vi "TableFinalizerRole.vi"(6 "Tactic index in":i32, 7 "first call":bool, 8 "error in (no error)":errorcluster, 10 "Game in":refnum<class "Game.lvclass">, 11 "TableFinalizerRole in":refnum<class "TableFinalizerRole.lvclass">) -> (0 "error out":errorcluster, 1 "tactic index":i32, 2 "Robot out":refnum<class "Robot.lvclass">, 3 "TableFinalizerRole out":refnum<class "TableFinalizerRole.lvclass">)   [LabVIEW 2023, in "TableFinalizerRole.lvclass"]
uses:
  TableFinalizerRole.lvclass
  Game_class/Game.lvclass
  Robot_class/Robot.lvclass
  Role_class/Role.lvclass/Role.ctl
  TableFinalizerRole.lvclass/TableFinalizerRole.ctl
  Tacticbook_class/Tacticbook.lvclass/Tacticbook.ctl
  TableReceiverTactic_class/TableReceiverTactic.lvclass/TableReceiverTactic.ctl
  ShootTactic_class/States.ctl
  ShootTactic_class/ShootTactic.lvclass/ShootTactic.ctl
  Tacticbook_class/Read TableReceiverTactic.vi
  TableReceiverTactic_class/Read States.vi
  Tacticbook_class/Write TableReceiverTactic.vi
  Tacticbook_class/Read WaitPassTactic.vi
  Tacticbook_class/Write WaitPassTactic.vi
  Tacticbook_class/Read ShootTactic.vi
  ShootTactic_class/Read States.vi
  Tacticbook_class/Write ShootTactic.vi
  Role_class/Read Tacticbook.vi
  Read number_of_tactics.vi
  Role_class/Write Tacticbook.vi
  Role_class/Write tactic_index.vi
  Role_class/Read RobotRef.vi
  Tacticbook_class/Tacticbook.lvclass
  KickToPassReceiverTactic_class/KickToPassReceiverTactic.lvclass
  TableReceiverTactic_class/TableReceiverTactic.lvclass
  WaitPassTactic_class/WaitPassTactic.lvclass
  ShootTactic_class/ShootTactic.lvclass
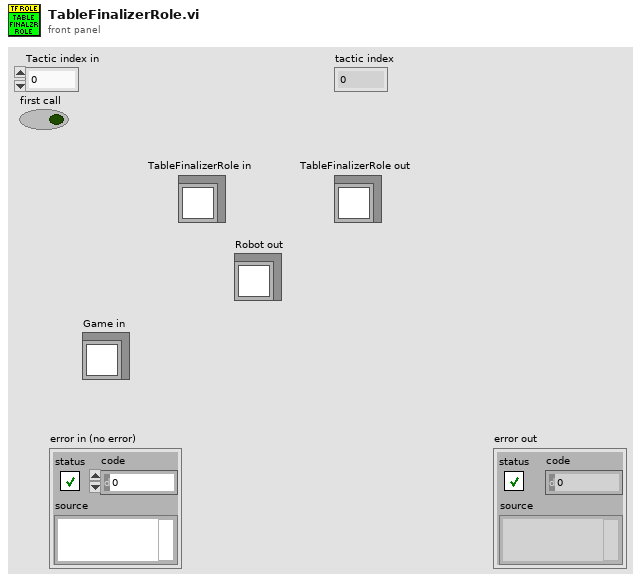
[diagram p1: front panel]
types:
  T1 = typedef "ShootTactic.lvclass/States.ctl" = enum16{"BallInGoalieArea", "Exit", "KickToGoal", "StealBall"}
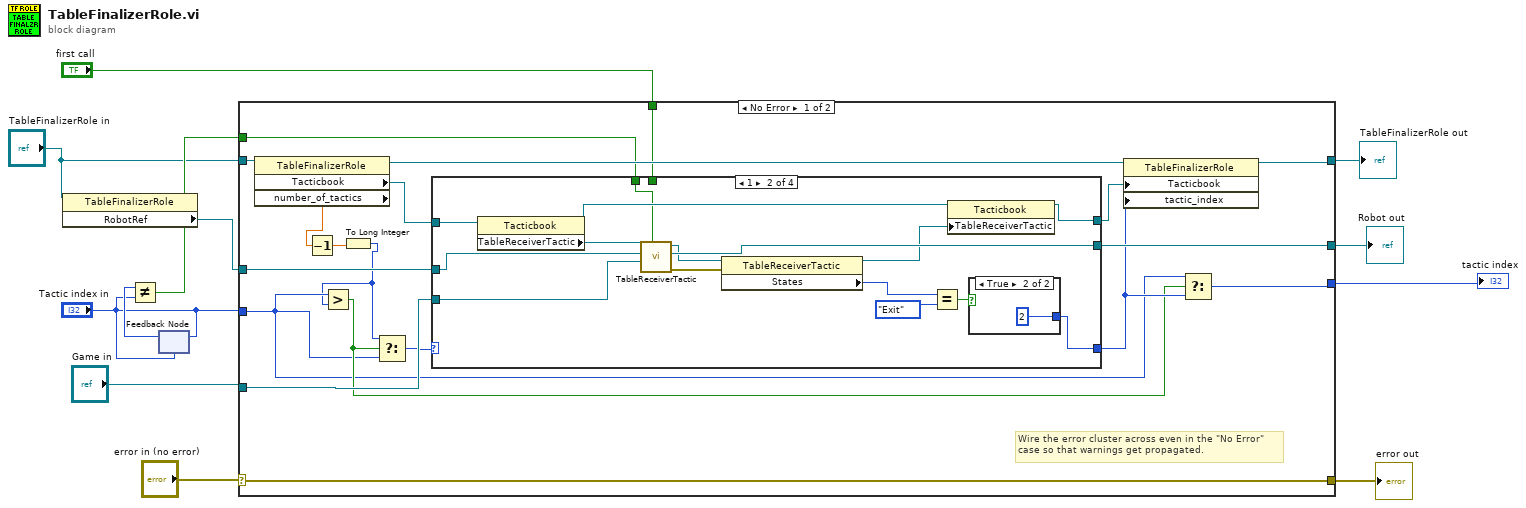
[diagram p0: block diagram]
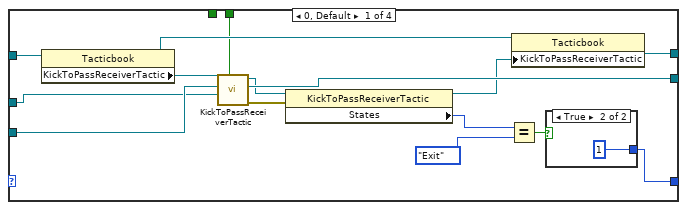
[diagram p2: hidden frame]
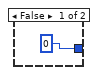
[diagram p3: hidden frame]
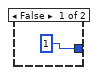
[diagram p4: hidden frame]
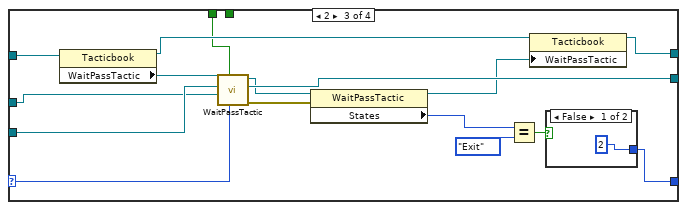
[diagram p5: hidden frame]
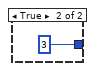
[diagram p6: hidden frame]
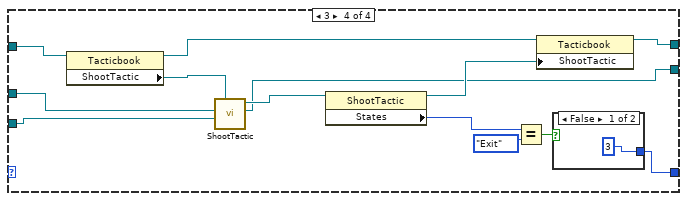
[diagram p7: hidden frame]
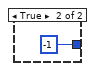
[diagram p8: hidden frame]
diagram:
  n1 = property class="TableFinalizerRole"(reference="TableFinalizerRole in") -> ("RobotRef"=w10:refnum<class "Robot.lvclass">)  [unwired: 1 in, 2 out]
  n2 = feedback #1("Tactic index in") -> (w6:i32)
  n3 = Not Equal?(x=w6, y="Tactic index in") -> (x != y?=w4:bool)
  n4 = feedback-in #1("Tactic index in") -> ()
  n5 = case shown="No Error" "error in (no error)" {
    selector: "error in (no error)" -> [w31 w101]
    tunnel: [w31 w101] -> w11
    tunnel: [w29 w100] -> w1
    tunnel: "TableFinalizerRole in" -> [w30 w100]
    tunnel: w10 -> [w26 w99]
    tunnel: [w25 w99] -> w3
    tunnel: "Game in" -> [w23 _]
    tunnel: [w21 _] -> w9
    tunnel: "Tactic index in" -> [w18 _]
    tunnel: "first call" -> [w16 _]
    tunnel: w4 -> [w13 _]
    frame No Error {
      # "Wire the error cluster across even in the \"No Error\"\ncase so that warnings get propagated."
      n6 = property class="TableFinalizerRole"(reference=w30) -> (reference out=w28:refnum<class "TableFinalizerRole.lvclass">, "Tacticbook"=w27:refnum<class "Tacticbook.lvclass">, "number_of_tactics"=w17:dbl)  [unwired: 1 in, 1 out]
      n7 = Decrement(x=w17) -> (x-1=w15:dbl)
      n8 = To Long Integer(number=w15) -> (32bit integer=w14:i32)
      n9 = Greater?(x=w18, y=w14) -> (0:w19:bool)
      n10 = Select(t=w14, s=w19, f=w18) -> (s? t:f=w20:i32)
      n11 = case shown="1" w20 {
        selector: w20 -> [_ _ w66 _]
        tunnel: [w34 w51 w69 w85] -> w22
        tunnel: w27 -> [w46 w63 w81 w94]
        tunnel: w26 -> [w37 w54 w72 w87]
        tunnel: [w45 w62 w80 w88] -> w25
        tunnel: [w41 w58 w76 w92] -> w24
        tunnel: w23 -> [w38 w55 w73 w86]
        tunnel: w16 -> [w32 _ _ _]
        tunnel: w13 -> [_ w49 w68 _]
        frame 0, Default {
          n12 = property class="Tacticbook"(reference=w46) -> (reference out=w43:refnum<class "Tacticbook.lvclass">, "KickToPassReceiverTactic"=w40:refnum<class "KickToPassReceiverTactic.lvclass">)  [unwired: 1 in, 1 out]
          n13 = call "KickToPassReceiverTactic.vi"("first call"=w32, "Robot"=w37, "Game in"=w38, "KickToPassReceiverTactic in"=w40) -> ("error out"=w44:errorcluster, "Robot out"=w45:refnum<class "Robot.lvclass">, "KickToPassReceiverTactic out"=w39:refnum<class "KickToPassReceiverTactic.lvclass">)  [unwired: 5 in]
          n14 = property class="KickToPassReceiverTactic"(reference=w39, error in=w44) -> (reference out=w42:refnum<class "KickToPassReceiverTactic.lvclass">, "States"=w35:enum16{"KickToPassReceiver", "WaitPass", "Exit"})  [unwired: 1 out]
          n15 = Equal?(x=w35, y=enum16{"KickToPassReceiver", "WaitPass", "Exit"}."Exit") -> (x = y?=w36:bool)
          n16 = property class="Tacticbook"(reference=w43, "KickToPassReceiverTactic"=w42) -> (reference out=w41:refnum<class "Tacticbook.lvclass">)  [unwired: 1 in, 1 out]
          n17 = case shown="True" w36 {
            tunnel: [0 1] -> w34
            frame False {
            }
            frame True {
            }
          }
        }
        frame 1 {
          n18 = property class="Tacticbook"(reference=w63) -> (reference out=w60:refnum<class "Tacticbook.lvclass">, "TableReceiverTactic"=w57:refnum<class "TableReceiverTactic.lvclass">)  [unwired: 1 in, 1 out]
          n19 = call "TableReceiverTactic.vi"("Firstcall?"=w49, "Game in"=w55, "Robot"=w54, "TableReceiverTactic in"=w57) -> ("error out"=w61:errorcluster, "Robot out"=w62:refnum<class "Robot.lvclass">, "TableReceiverTactic out"=w56:refnum<class "TableReceiverTactic.lvclass">)  [unwired: 5 in]
          n20 = property class="TableReceiverTactic"(reference=w56, error in=w61) -> (reference out=w59:refnum<class "TableReceiverTactic.lvclass">, "States"=w52:enum16{"Halt", "Exit", "GoTo"})  [unwired: 1 out]
          n21 = Equal?(x=w52, y=enum16{"Halt", "Exit", "GoTo"}."Exit") -> (x = y?=w53:bool)
          n22 = property class="Tacticbook"(reference=w60, "TableReceiverTactic"=w59) -> (reference out=w58:refnum<class "Tacticbook.lvclass">)  [unwired: 1 in, 1 out]
          n23 = case shown="True" w53 {
            tunnel: [1 2] -> w51
            frame False {
            }
            frame True {
            }
          }
        }
        frame 2 {
          n24 = property class="Tacticbook"(reference=w81) -> (reference out=w78:refnum<class "Tacticbook.lvclass">, "WaitPassTactic"=w75:refnum<class "WaitPassTactic.lvclass">)  [unwired: 1 in, 1 out]
          n25 = call-dynamic "WaitPassTactic.vi"("Tactic index in"=w66, "first call"=w68, "Robot"=w72, "Game in"=w73, "WaitPassTactic in"=w75) -> ("error out"=w79:errorcluster, "Robot out"=w80:refnum<class "Robot.lvclass">, "WaitPassTactic out"=w74:refnum<class "WaitPassTactic.lvclass">)  [unwired: 4 in]
          n26 = property class="WaitPassTactic"(reference=w74, error in=w79) -> (reference out=w77:refnum<class "WaitPassTactic.lvclass">, "States"=w70:enum16{"State 0", "State 1", "State 2", "Exit"})  [unwired: 1 out]
          n27 = Equal?(x=w70, y=enum16{"State 0", "State 1", "State 2", "Exit"}."Exit") -> (x = y?=w71:bool)
          n28 = property class="Tacticbook"(reference=w78, "WaitPassTactic"=w77) -> (reference out=w76:refnum<class "Tacticbook.lvclass">)  [unwired: 1 in, 1 out]
          n29 = case shown="False" w71 {
            tunnel: [2 3] -> w69
            frame False {
            }
            frame True {
            }
          }
        }
        frame 3 {
          n30 = property class="Tacticbook"(reference=w94) -> (reference out=w93:refnum<class "Tacticbook.lvclass">, "ShootTactic"=w90:refnum<class "ShootTactic.lvclass">)  [unwired: 1 in, 1 out]
          n31 = call "ShootTactic.vi"("Game in"=w86, "Robot"=w87, "ShootTactic in"=w90) -> ("Robot out"=w88:refnum<class "Robot.lvclass">, "ShootTactic out"=w89:refnum<class "ShootTactic.lvclass">)  [unwired: 6 in, 1 out]
          n32 = property class="ShootTactic"(reference=w89) -> (reference out=w91:refnum<class "ShootTactic.lvclass">, "States"=w95:T1)  [unwired: 1 in, 1 out]
          n33 = Equal?(x=w95, y=States."Exit") -> (x = y?=w96:bool)
          n34 = property class="Tacticbook"(reference=w93, "ShootTactic"=w91) -> (reference out=w92:refnum<class "Tacticbook.lvclass">)  [unwired: 1 in, 1 out]
          n35 = case shown="False" w96 {
            tunnel: [3 -1] -> w85
            frame False {
            }
            frame True {
            }
          }
        }
      }
      n36 = property class="TableFinalizerRole"(reference=w28, "Tacticbook"=w24, "tactic_index"=w22) -> (reference out=w29:refnum<class "TableFinalizerRole.lvclass">)  [unwired: 1 in, 1 out]
      n37 = Select(t=w18, s=w19, f=w22) -> (s? t:f=w21:i32)
    }
    frame Error {
    }
  }
  "error out" <- w11
  "tactic index" <- w9
  "Robot out" <- w3
  "TableFinalizerRole out" <- w1
